vi "Format Audio For Output.vi"(10 "Headphone Audio":dbl[][](array[numeric]), 11 "Master Audio":dbl[][](array[numeric])) -> (3 "Audio Output":T1)   [LabVIEW 2020, in "Audio Output.lvlib"]
uses:
  Audio Output.lvlib
  Audio Output Queue Type.ctl
  Packed Libraries/Audio Processing.lvlibp
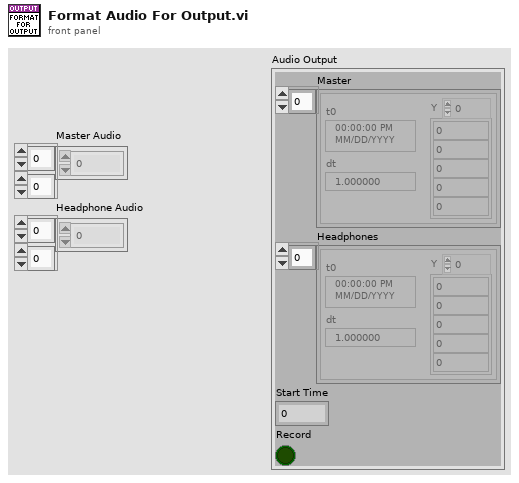
[diagram p1: front panel]
types:
  T1 = typedef "Audio Output.lvlib/Audio Output Queue Type.ctl" = cluster{"Master":waveform(i16)[], "Headphones":waveform(i16)[], "Start Time":dbl, "Record":bool}
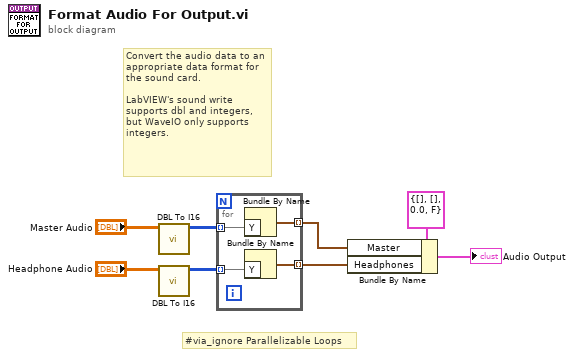
[diagram p0: block diagram]
diagram:
  # "#via_ignore Parallelizable Loops"
  # "Convert the audio data to an appropriate data format for the sound card.\n\nLabVIEW's sound write supports dbl and integers, but WaveIO only supports integers."
  n1 = call "DBL To I16.vi"("Audio Data (2D DBL)"="Master Audio") -> ("Audio Data (2D I16)"=w5:i16[][])  [unwired: 9 in, 1 out]
  n2 = call "DBL To I16.vi"("Audio Data (2D DBL)"="Headphone Audio") -> ("Audio Data (2D I16)"=w4:i16[][])  [unwired: 9 in, 1 out]
  n3 = for {
    tunnel: w5 -> [w12] mode=indexing
    tunnel: [w11] -> w7 mode=indexing
    tunnel: w4 -> [w10] mode=indexing
    tunnel: [w9] -> w6 mode=indexing
    n4 = Bundle By Name("Y"=w12) -> (w11:waveform(i16))  [unwired: 1 in]
    n5 = Bundle By Name("Y"=w10) -> (w9:waveform(i16))  [unwired: 1 in]
  }
  n6 = Bundle By Name(cluster=T1 {"Master"=[], "Headphones"=[], "Start Time"=0.0, "Record"=FALSE}, "Master"=w7, "Headphones"=w6) -> (→"Audio Output":T1)
